vi "Read Output Conversion.vi"(10 "Process Data Input":u8[](array[numeric]), 11 "Drives":T1(array[cluster])) -> (3 "Map":map{string, dbl}(c390))   [LabVIEW 2024, in "EtherCAT Model.lvlib"]
uses:
  EtherCAT Model.lvlib
  <instrlib>/_Ackermann Automation/EtherCAT Lib/EcatLib/EthercatLib.lvlib
  <instrlib>/_Ackermann Automation/EtherCAT Lib/EcatLib/Conversion/ConvertFrameToBoolean.vi
  <instrlib>/_Ackermann Automation/EtherCAT Lib/EcatLib/Conversion/ConvertFrameToU16.vi
  <instrlib>/_Ackermann Automation/EtherCAT Lib/EcatLib/Conversion/ConvertFrameToI16.vi
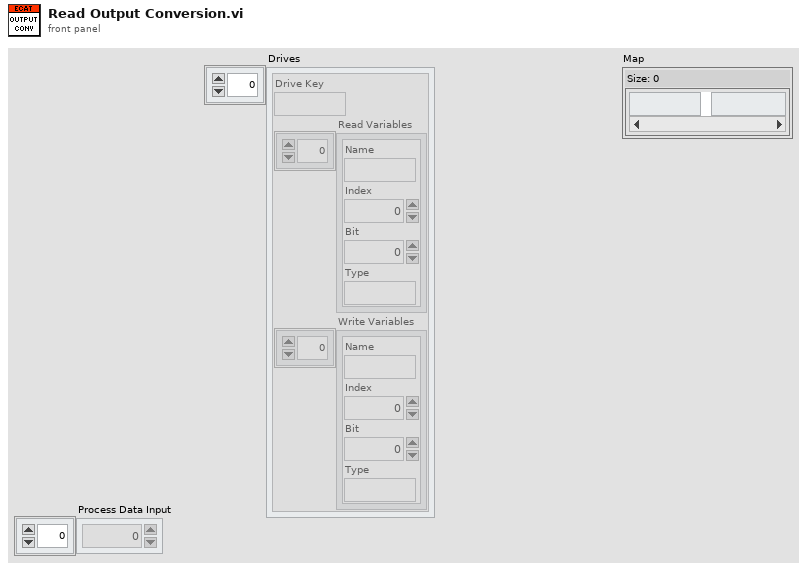
[diagram p1: front panel]
types:
  T1 = cluster{"Drive Key":string, "Read Variables":cluster{"Name":string, "Index":i32, "Bit":u8, "Type":string}[], "Write Variables":cluster{"Name":string, "Index":i32, "Bit":u8, "Type":string}[]}[]
  T2 = cluster{"Name":string, "Index":i32, "Bit":u8, "Type":string}[]
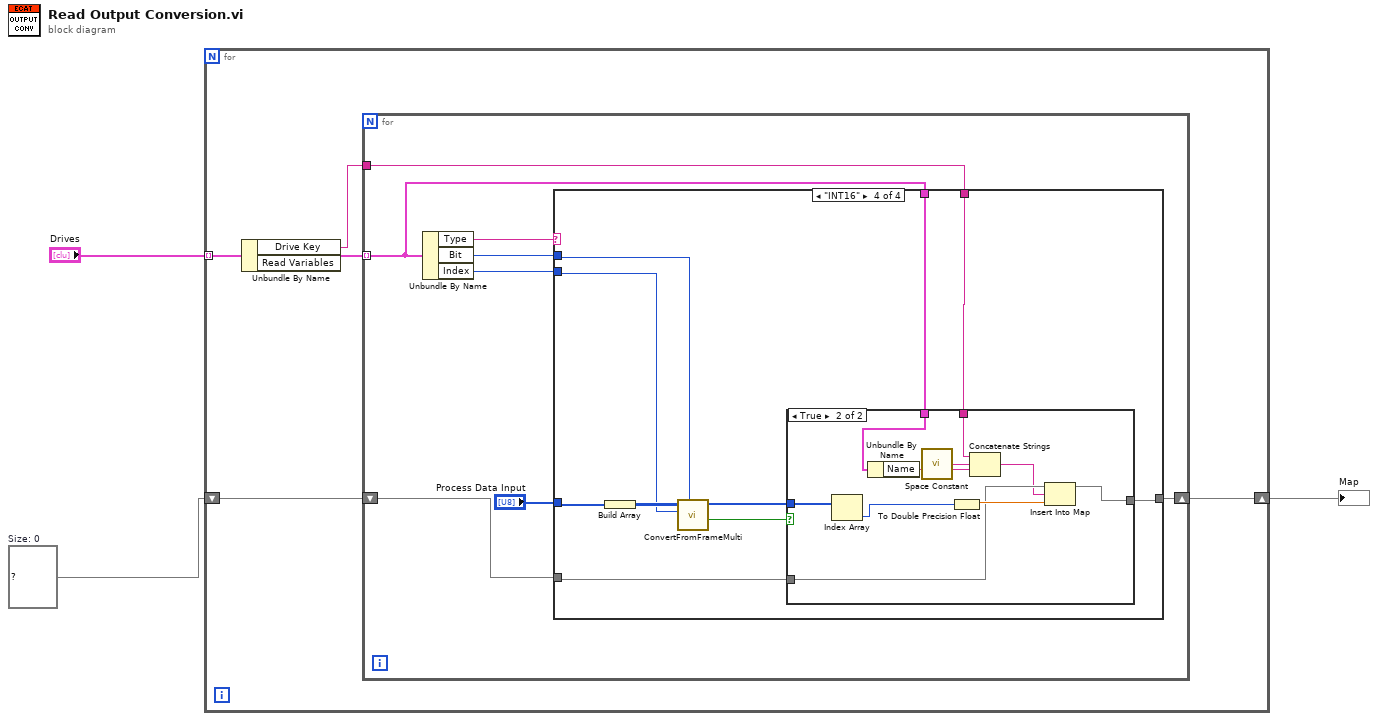
[diagram p0: block diagram]
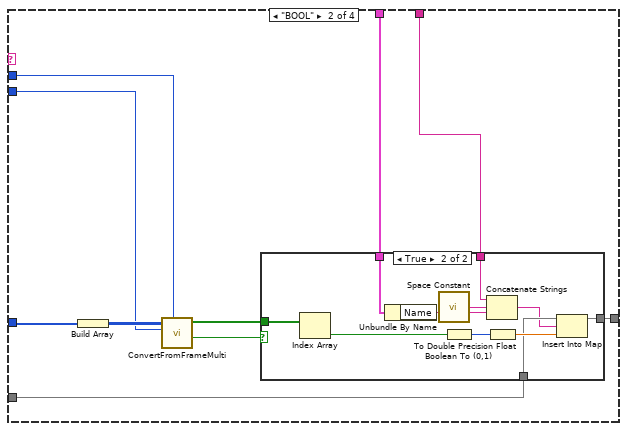
[diagram p3: hidden frame]
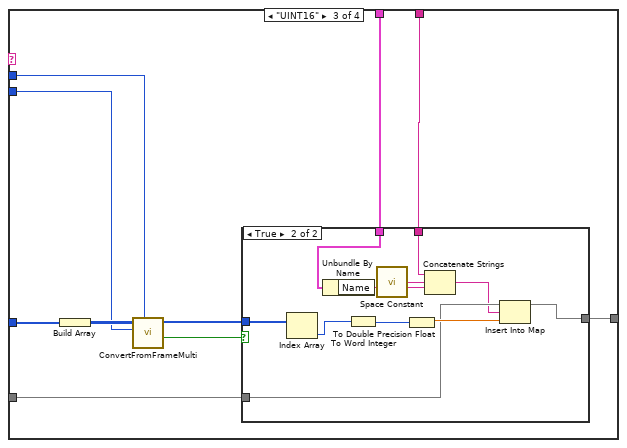
[diagram p5: hidden frame]
diagram:
  w2 = map{string, dbl} {}  # Size: 0
  n1 = for {
    tunnel: "Drives" -> [w8] mode=indexing
    shift-right: [w4] -> w1
    shift-left: w2 -> [w6]
    n2 = Unbundle By Name(w8) -> ("Drive Key"=w5:string, "Read Variables"=w7:T2)
    n3 = for {
      tunnel: w7 -> [w11] mode=indexing
      tunnel: w5 -> [w10]
      shift-right: [w9] -> w4
      shift-left: w6 -> [w12]
      n4 = Unbundle By Name(w11) -> ("Type"=w16:string, "Bit"=w13:u8, "Index"=w14:i32)
      n5 = case shown="\"INT16\"" w16 {
        tunnel: "Process Data Input" -> [_ w27 w49 w64]
        tunnel: w14 -> [_ w25 w47 w65]
        tunnel: w13 -> [_ w24 w46 w66]
        tunnel: w12 -> [w17 w21 w43 w63]
        tunnel: w11 -> [_ w20 w41 w67]
        tunnel: w10 -> [_ w19 w40 w68]
        tunnel: [w17 w18 w44 w62] -> w9
        frame Default {
        }
        frame "BOOL" {
          n6 = Build Array(w27) -> (w26:u8[][])
          n7 = call-poly <instrlib>:"ConvertFromFrameMulti.vi"("Bit Index"=w24, "Byte Index"=w25, "Acquisition Data"=w26) -> ("Output Data Valid"=w23:bool, "Bit"=w22:bool[])  [unwired: 7 in]
          n8 = case shown="True" w23 {
            tunnel: w22 -> [_ w39]
            tunnel: w21 -> [w28 w35]
            tunnel: w20 -> [_ w34]
            tunnel: w19 -> [_ w31]
            tunnel: [w28 w29] -> w18
            frame False {
            }
            frame True {
              n9 = Index Array(array=w39) -> (element=w38:bool)  [unwired: 1 in]
              n10 = Unbundle By Name(w34) -> ("Name"=w33:string)
              n11 = call <vilib>:"Space Constant.vi"() -> ("String"=w32:string)
              n12 = Boolean To (0,1)(Boolean=w38) -> (0, 1=w37:i16)
              n13 = Concatenate Strings(w31, w32, w33) -> (w30:string)
              n14 = To Double Precision Float(number=w37) -> (double precision float=w36:dbl)
              n15 = Insert Into Map(map in=w35, key=w30, value=w36) -> (map out=w29:map{string, dbl})  [unwired: 2 out]
            }
          }
        }
        frame "UINT16" {
          n16 = Build Array(w49) -> (w48:u8[][])
          n17 = call-poly <instrlib>:"ConvertFromFrameMulti.vi"("Bit Index"=w46, "Byte Index"=w47, "Acquisition Data"=w48) -> ("Output Data Valid"=w45:bool, "U16"=w42:u16[])  [unwired: 7 in]
          n18 = case shown="True" w45 {
            tunnel: [w50 w57] -> w44
            tunnel: w43 -> [w50 w56]
            tunnel: w42 -> [_ w60]
            tunnel: w41 -> [_ w53]
            tunnel: w40 -> [_ w52]
            frame False {
            }
            frame True {
              n19 = Index Array(array=w60) -> (element=w59:u16)  [unwired: 1 in]
              n20 = Unbundle By Name(w53) -> ("Name"=w55:string)
              n21 = To Word Integer(number=w59) -> (16bit integer=w61:i16)
              n22 = call <vilib>:"Space Constant.vi"() -> ("String"=w54:string)
              n23 = To Double Precision Float(number=w61) -> (double precision float=w58:dbl)
              n24 = Concatenate Strings(w52, w54, w55) -> (w51:string)
              n25 = Insert Into Map(map in=w56, key=w51, value=w58) -> (map out=w57:map{string, dbl})  [unwired: 2 out]
            }
          }
        }
        frame "INT16" {
          n26 = Build Array(w64) -> (w71:u8[][])
          n27 = call-poly <instrlib>:"ConvertFromFrameMulti.vi"("Bit Index"=w66, "Byte Index"=w65, "Acquisition Data"=w71) -> ("Output Data Valid"=w70:bool, "I16"=w69:i16[])  [unwired: 7 in]
          n28 = case shown="True" w70 {
            tunnel: [w72 w79] -> w62
            tunnel: w63 -> [w72 w78]
            tunnel: w69 -> [_ w82]
            tunnel: w67 -> [_ w75]
            tunnel: w68 -> [_ w74]
            frame False {
            }
            frame True {
              n29 = Index Array(array=w82) -> (element=w81:i16)  [unwired: 1 in]
              n30 = Unbundle By Name(w75) -> ("Name"=w77:string)
              n31 = call <vilib>:"Space Constant.vi"() -> ("String"=w76:string)
              n32 = To Double Precision Float(number=w81) -> (double precision float=w80:dbl)
              n33 = Concatenate Strings(w74, w76, w77) -> (w73:string)
              n34 = Insert Into Map(map in=w78, key=w73, value=w80) -> (map out=w79:map{string, dbl})  [unwired: 2 out]
            }
          }
        }
      }
    }
  }
  "Map" <- w1
